vi "写入湿度数据.vi"(0 "表格控件":string[][](table)) -> ()   [LabVIEW 2012]
doc: "本VI通过将表格写入Excel工作表说明利用OLE自动化VI的基本方式。"
panel:
  in  "Completion Task":u16(ring) caption="完成任务" items=["保持Excel打开", "关闭电子表格"]
  out "error out":errorcluster caption="错误输出"
  in  "error in (no error)":errorcluster caption="错误输入（无错误）"
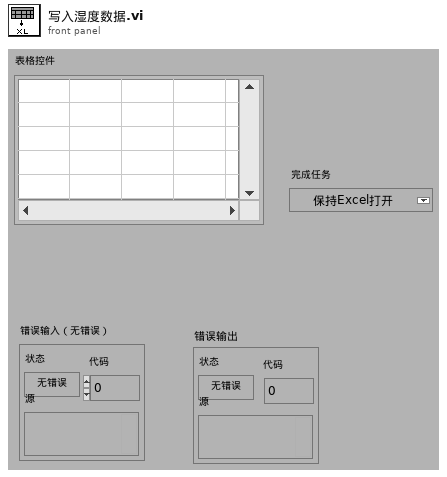
[diagram p1: front panel]
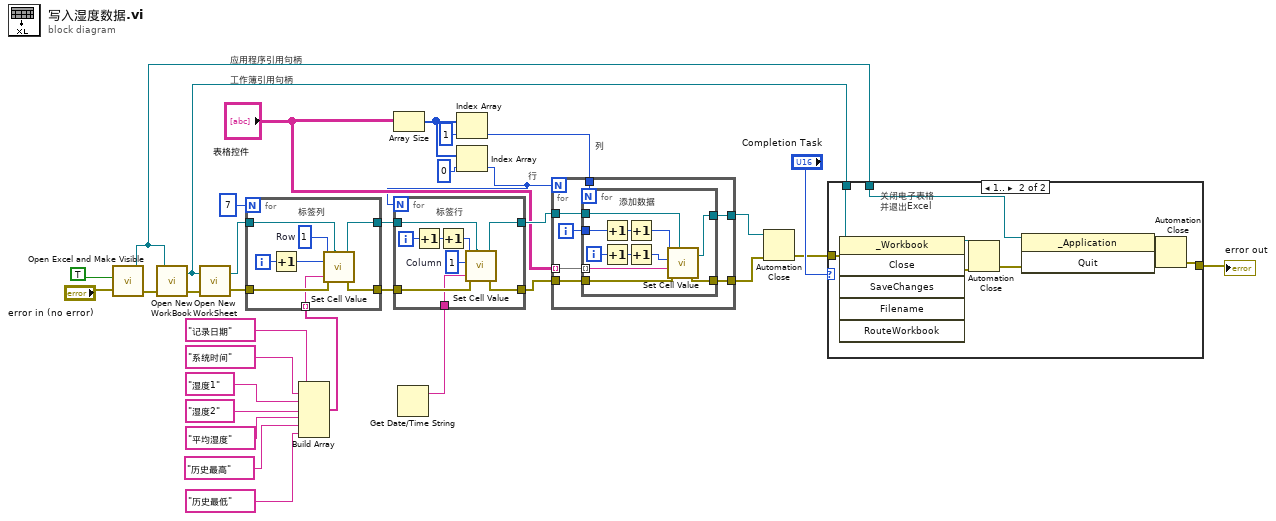
[diagram p0: block diagram]
diagram:
  # "列"
  # "行"
  # "工作簿引用句柄"
  # "应用程序引用句柄"
  n1 = call "Open Excel and Make Visible.vi"("error in (no error)"="error in (no error)", "Visible Boolean"=TRUE) -> ("error out"=w28:errorcluster, "Excel._Application"=w23:refnum<k7>)
  n2 = call "Open New  WorkBook.vi"("error in (no error)"=w28, "Excel._Application"=w23) -> ("error out"=w27:errorcluster, "Excel._Workbook"=w24:refnum<k7>)  [unwired: 1 out]
  n3 = call "Open New WorkSheet.vi"("error in (no error)"=w27, "Excel._Workbook"=w24) -> ("error out"=w18:errorcluster, "Excel._Worksheet"=w19:refnum<k7>)  [unwired: 1 out]
  n4 = Build Array("记录日期", "系统时间", "湿度1", "湿度2", "平均湿度", "历史最高", "历史最低") -> (w14:string[])
  n5 = for {
    N: 7 -> [_]
    tunnel: w19 -> [w40]
    tunnel: w18 -> [w39]
    tunnel: [w38] -> w12
    tunnel: [w37] -> w10
    tunnel: w14 -> [w35] mode=indexing
    i -> [w41]
    w36 = 1  # Row
    # "标签列"
    n6 = Increment(x=w41) -> (x+1=w34:i32)
    n7 = call "Set Cell Value.vi"("Row"=w36, "Col"=w34, "Value"=w35, "error in (no error)"=w39, "Excel._Worksheet"=w40) -> ("Excel._Worksheet"=w37:refnum<k7>, "error out"=w38:errorcluster)
  }
  n8 = Array Size(array="表格控件") -> (size(s)=w33:i32[])
  n9 = Get Date/Time String() -> (date string=w8:string)  [unwired: 3 in, 1 out]
  n10 = Index Array(array=w33, index=1) -> (element=w26:i32)
  n11 = Index Array(array=w33, index=0) -> (element=w1:i32)
  n12 = for {
    N: w1 -> [_]
    tunnel: w10 -> [w46]
    tunnel: w12 -> [w45]
    tunnel: [w44] -> w11
    tunnel: [w43] -> w9
    tunnel: w8 -> [w42]
    i -> [w50]
    w48 = 1  # Column
    # "标签行"
    n13 = Increment(x=w50) -> (x+1=w49:i32)
    n14 = Increment(x=w49) -> (x+1=w47:i32)
    n15 = call "Set Cell Value.vi"("Row"=w47, "Col"=w48, "Value"=w42, "error in (no error)"=w45, "Excel._Worksheet"=w46) -> ("Excel._Worksheet"=w43:refnum<k7>, "error out"=w44:errorcluster)
  }
  n16 = for {
    N: w1 -> [_]
    tunnel: w9 -> [w57]
    tunnel: w11 -> [w55]
    tunnel: [w56] -> w22
    tunnel: "表格控件" -> [w54] mode=indexing
    tunnel: w26 -> [w53]
    tunnel: [w52] -> w20
    i -> [w51]
    n17 = for {
      N: w53 -> [_]
      tunnel: w57 -> [w64]
      tunnel: w55 -> [w63]
      tunnel: [w62] -> w56
      tunnel: w51 -> [w61]
      tunnel: w54 -> [w60] mode=indexing
      tunnel: [w59] -> w52
      i -> [w68]
      # "添加数据"
      n18 = Increment(x=w61) -> (x+1=w67:i32)
      n19 = Increment(x=w68) -> (x+1=w65:i32)
      n20 = Increment(x=w67) -> (x+1=w66:i32)
      n21 = Increment(x=w65) -> (x+1=w58:i32)
      n22 = call "Set Cell Value.vi"("Row"=w66, "Col"=w58, "Value"=w60, "error in (no error)"=w63, "Excel._Worksheet"=w64) -> ("Excel._Worksheet"=w59:refnum<k7>, "error out"=w62:errorcluster)
    }
  }
  n23 = Automation Close(3:w22, 5:w20) -> (0:w21:errorcluster)
  n24 = case shown="1.." "Completion Task" {
    tunnel: [w69 w70] -> w4
    tunnel: w24 -> [_ w78]
    tunnel: w23 -> [_ w74]
    tunnel: w21 -> [w69 w77]
    frame ..0 {
    }
    frame 1.. {
      # "关闭电子表格\n并退出Excel"
      n25 = invoke class="_Workbook" method="Close"(reference=w78, error in=w77) -> (reference out=w76:refnum<k7>, error out=w75:errorcluster)  [unwired: 4 in, 4 out]
      n26 = Automation Close(3:w75, 5:w76) -> (0:w73:errorcluster)
      n27 = invoke class="_Application" method="Quit"(reference=w74, error in=w73) -> (reference out=w71:refnum<k7>, error out=w72:errorcluster)  [unwired: 1 in, 1 out]
      n28 = Automation Close(3:w72, 5:w71) -> (0:w70:errorcluster)
    }
  }
  "error out" <- w4
